vi "Example Raspi Pico GPIO 1.vi"() -> ()   [LabVIEW 2014]
uses:
  LabVIEW Universal Transciptor Raspberry Pi Pico.lvlib
panel:
  in  "enabled":bool
  in  "num":u8
  in  "gpio 3":u32
  in  "value 2":bool
  in  "gpio 2":dbl
  in  "fn":u16(ring) items=["GPIO_FUNC_XIP"=0, "GPIO_FUNC_SPI"=1, "GPIO_FUNC_UART"=2, "GPIO_FUNC_I2C"=3, "GPIO_FUNC_PWM"=4, "GPIO_FUNC_SIO"=5, "GPIO_FUNC_PIO0"=6, "GPIO_FUNC_PIO1"=7, "GPIO_FUNC_GPCK"=8, "GPIO_FUNC_USB"=9, "GPIO_FUNC_NULL"=31]
  out "value":bool
  in  "gpio":u32
  out "Error Out":errorcluster
  in  "Error In":errorcluster
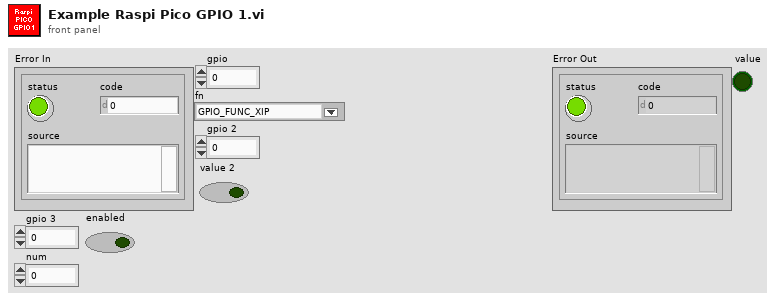
[diagram p1: front panel]
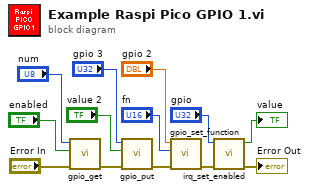
[diagram p0: block diagram]
diagram:
  n1 = call "gpio_get.vi"("num"="num", "enabled"="enabled", "Error In"="Error In") -> ("Error Out"=w9:errorcluster)  [unwired: 7 in]
  n2 = call "gpio_put.vi"("Error In"=w9, "value"="value 2", "gpio"="gpio 3") -> ("Error Out"=w10:errorcluster)  [unwired: 8 in]
  n3 = call "gpio_set_function.vi"("Error In"=w10, "fn"="fn", "gpio"="gpio 2") -> ("Error Out"=w11:errorcluster)  [unwired: 8 in]
  n4 = call "irq_set_enabled.vi"("gpio"="gpio", "Error In"=w11) -> ("value"=→"value":bool, "Error Out"=→"Error Out":errorcluster)  [unwired: 7 in]
